vi "encodeEnum.vi"(6 "MsgPack Config":T1={"Cluster Conversion"=enum."to array", "Enum Conversion"=enum."to uint", "Use ArrayType"=FALSE}, 8 "error in (no error)":errorcluster, 10 "Type":T4, 11 "Variant":variant) -> (0 "error out":errorcluster, 3 "Array":u8[](array[numeric]))   [LabVIEW 2016, in "MsgPack.lvlib"]
uses:
  MsgPack.lvlib
  <vilib>/Utility/Data Type/Type Definitions/Data Type.ctl
  SubVis/msgpack_config.ctl
  SubVis/cluster_conversion.ctl
  SubVis/enum_conversion.ctl
  <vilib>/Utility/Data Type/NI_Data Type.lvlib
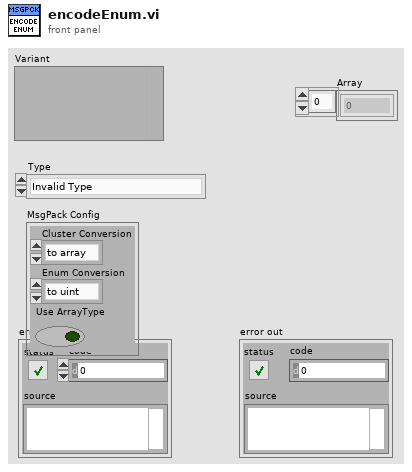
[diagram p1: front panel]
types:
  T1 = typedef "MsgPack.lvlib/msgpack_config.ctl" = cluster{"Cluster Conversion":T2, "Enum Conversion":T3, "Use ArrayType":bool}
  T2 = typedef "MsgPack.lvlib/cluster_conversion.ctl" = enum16{"to map", "to array"}
  T3 = typedef "MsgPack.lvlib/enum_conversion.ctl" = enum16{"to uint", "to string"}
  T4 = typedef "NI_Data Type.lvlib/Data Type.ctl" = enum8{"Invalid Type", "Void", "I8", "I16", "I32", "I64", "U8", "U16", "U32", "U64", "Single Float", "Double Float", "Extended Float", "Single Complex", "Double Complex", "Extended Complex", "Enum U8", "Enum U16", "Enum U32", "Enum U64", "Single Float With Unit", "Double Float With Unit", "Extended Float With Unit", "Single Complex with Unit", "Double Complex with Unit", "Extended Complex with Unit", "Boolean", "String", "Path", "Picture", "Tag", "Array", "Cluster", "Variant", "LV Variant", "Waveform", "Timestamp", "Digital Waveform", "Digital Data", "ExpressData", "Refnum", "External Data", "VI", "Poly VI", "LabVIEW Class Instance", "Fixed Point"}
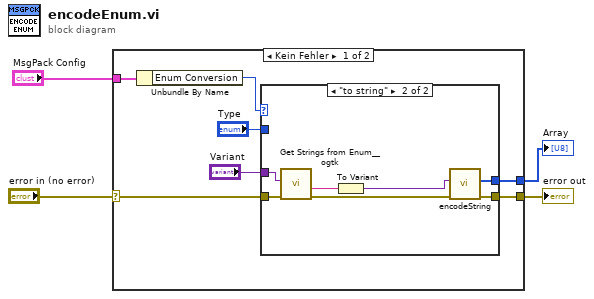
[diagram p0: block diagram]
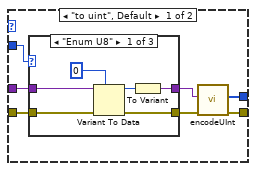
[diagram p2: hidden frame]
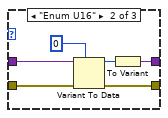
[diagram p3: hidden frame]
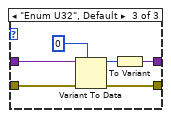
[diagram p4: hidden frame]
diagram:
  n1 = case shown="Kein Fehler" "error in (no error)" {
    selector: "error in (no error)" -> [w5 w44]
    tunnel: [w9 _] -> w4
    tunnel: [w8 w44] -> w3
    tunnel: "MsgPack Config" -> [w7 _]
    frame No Error {
      n2 = Unbundle By Name(w7) -> ("Enum Conversion"=w6:T3)
      n3 = case shown="\"to string\"" w6 {
        tunnel: [w18 w39] -> w8
        tunnel: [w17 w38] -> w9
        tunnel: w5 -> [w16 w42]
        tunnel: "Type" -> [w14 _]
        tunnel: "Variant" -> [w12 w37]
        frame "to uint", Default {
          n4 = case shown="\"Enum U8\"" w14 {
            tunnel: [w22 w28 w35] -> w13
            tunnel: w12 -> [w19 w25 w33]
            tunnel: w16 -> [w20 w26 w32]
            tunnel: [w21 w27 w31] -> w15
            frame "Enum U8" {
              n5 = Variant To Data(error in=w20, type=u8 0, Variant=w19) -> (data=w24:u8, error out=w21:errorcluster)
              n6 = To Variant(anything=w24) -> (Variant=w22:variant)
            }
            frame "Enum U16" {
              n7 = Variant To Data(error in=w26, type=u16 0, Variant=w25) -> (data=w29:u16, error out=w27:errorcluster)
              n8 = To Variant(anything=w29) -> (Variant=w28:variant)
            }
            frame "Enum U32", Default {
              n9 = Variant To Data(error in=w32, type=u32 0, Variant=w33) -> (data=w36:u32, error out=w31:errorcluster)
              n10 = To Variant(anything=w36) -> (Variant=w35:variant)
            }
          }
          n11 = call "encodeUInt.vi"("error in (no error)"=w15, "Variant"=w13) -> ("error out"=w18:errorcluster, "Array"=w17:u8[])  [unwired: 8 in]
        }
        frame "to string" {
          n12 = call <userlib>:"Get Strings from Enum__ogtk.vi"("error in (no error)"=w42, "Enum"=w37) -> ("error out"=w40:errorcluster, "String Value"=w43:string)  [unwired: 6 in, 2 out]
          n13 = To Variant(anything=w43) -> (Variant=w41:variant)
          n14 = call "encodeString.vi"("error in (no error)"=w40, "Variant"=w41) -> ("error out"=w39:errorcluster, "Array"=w38:u8[])  [unwired: 8 in]
        }
      }
    }
    frame Error {
    }
  }
  "Array" <- w4
  "error out" <- w3
